vi "Sampled Data.vi"(8 "Error In":errorcluster, 10 "Data Sample":dbl, 11 "refnum in":refnum<file>) -> (0 "error out":errorcluster, 3 "refnum out":refnum<file>)   [LabVIEW 2018]
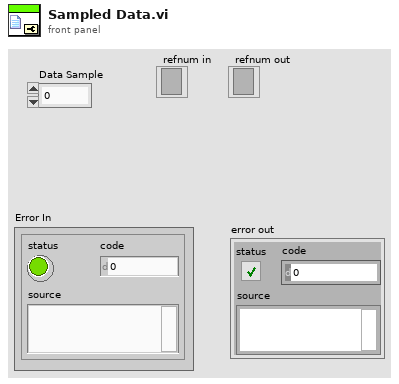
[diagram p1: front panel]
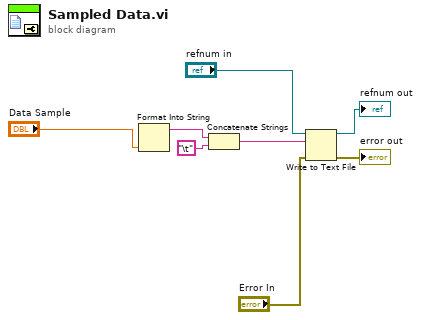
[diagram p0: block diagram]
diagram:
  n1 = Format Into String "Format Into String"("Data Sample") -> (resulting string=w1:string)  [unwired: 3 in, 1 out]
  n2 = Concatenate Strings(w1, "\t") -> (w3:string)
  n3 = Write to Text File(file (use dialog)="refnum in", text=w3, error in="Error In") -> (refnum out=→"refnum out":refnum<file>, error out=→"error out":errorcluster)  [unwired: 1 in, 1 out]
